vi "GetWiringType.vi"(11 "channels":T1[](array[typedef])) -> (3 "delta connection?":bool)   [LabVIEW 2017, in "McsaFpgaAcquisition.lvlib"]
uses:
  <vilib>/addons/InsightCM/Devices/Shared/Mcsa/McsaFpgaAcquisition/McsaFpgaAcquisition.lvlib
  <vilib>/addons/InsightCM/MessageBus/Base/controls/R2_Channel.ctl
  <vilib>/addons/InsightCM/MessageBus/Base/controls/KeyValuePair.ctl
  <vilib>/addons/InsightCM/MessageBus/Base/controls/Metric.ctl
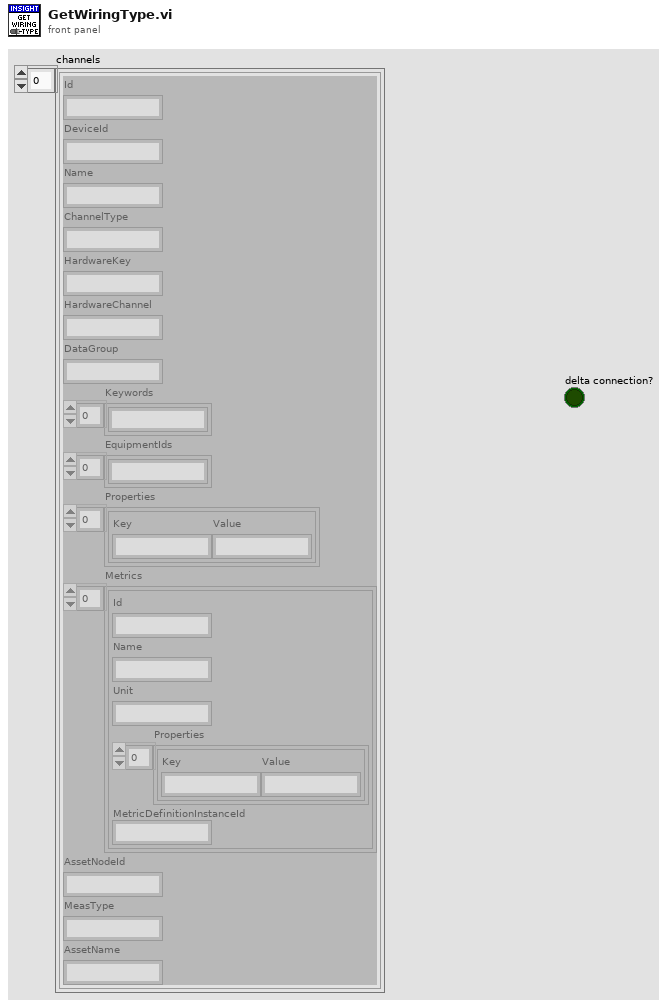
[diagram p1: front panel]
types:
  T1 = typedef "R2_Channel.ctl" = cluster{"Id":string, "DeviceId":string, "Name":string, "ChannelType":string, "HardwareKey":string, "HardwareChannel":string, "DataGroup":string, "Keywords":string[], "EquipmentIds":string[], "Properties":T2[], "Metrics":T3[], "AssetNodeId":string, "MeasType":string, "AssetName":string}
  T2 = typedef "KeyValuePair.ctl" = cluster{"Key":string, "Value":string}
  T3 = typedef "Metric.ctl" = cluster{"Id":string, "Name":string, "Unit":string, "Properties":T2[], "MetricDefinitionInstanceId":string}
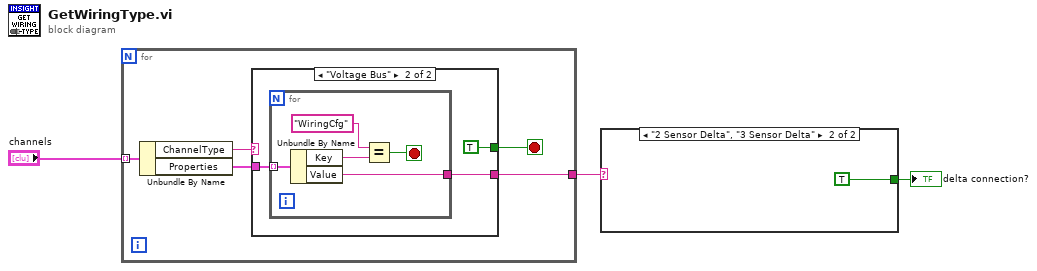
[diagram p0: block diagram]
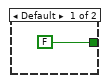
[diagram p2: hidden frame]
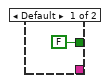
[diagram p3: hidden frame]
diagram:
  n1 = for {
    tunnel: "channels" -> [w8] mode=indexing
    tunnel: [w5] -> w2
    stop <- w4 stop-if-true
    n2 = Unbundle By Name(w8) -> ("ChannelType"=w7:string, "Properties"=w6:T2[])
    n3 = case shown="\"Voltage Bus\"" w7 {
      tunnel: w6 -> [_ w12]
      tunnel: [_ w11] -> w5
      tunnel: [FALSE TRUE] -> w4
      frame Default {
      }
      frame "Voltage Bus" {
        n4 = for {
          tunnel: w12 -> [w17] mode=indexing
          tunnel: [w13] -> w11
          stop <- w14 stop-if-true
          n5 = Unbundle By Name(w17) -> ("Key"=w16:string, "Value"=w13:string)
          n6 = Equal?(x="WiringCfg", y=w16) -> (x = y?=w14:bool)
        }
      }
    }
  }
  n7 = case shown="\"2 Sensor Delta\", \"3 Sensor Delta\"" w2 {
    tunnel: [FALSE TRUE] -> w1
    frame Default {
    }
    frame "2 Sensor Delta", "3 Sensor Delta" {
    }
  }
  "delta connection?" <- w1
